vi "_PC_Pub_check_numstr.vi"(4 "ValueType":enum16{"Double", "Unsign Int32", "Sign Int32"}(ring), 7 "NumStringIn":string) -> (0 "DBL output":dbl, 1 "I64 output":i64, 2 "Error?":bool, 3 "NumStringOut":string)   [LabVIEW 2018]
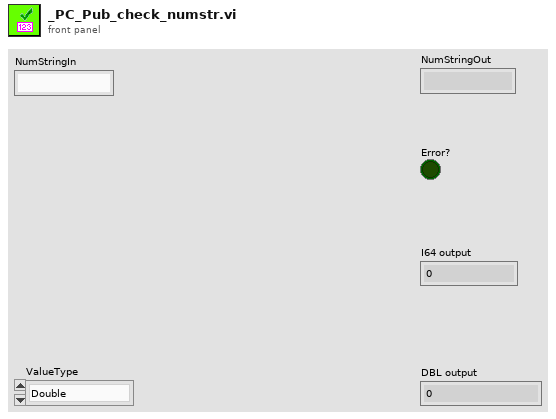
[diagram p1: front panel]
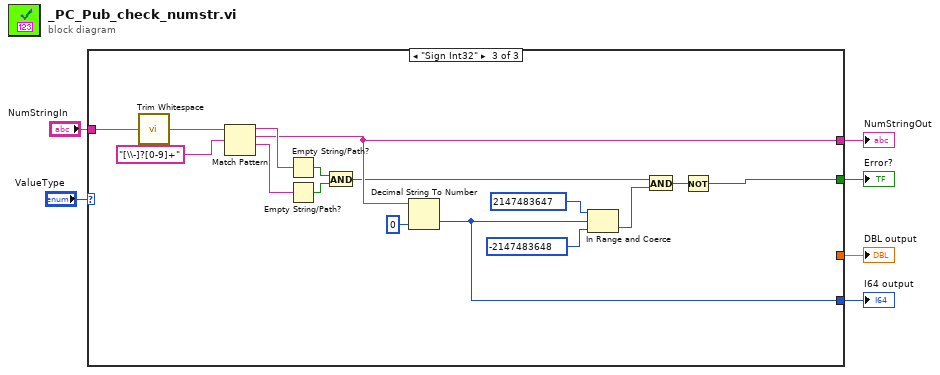
[diagram p0: block diagram]
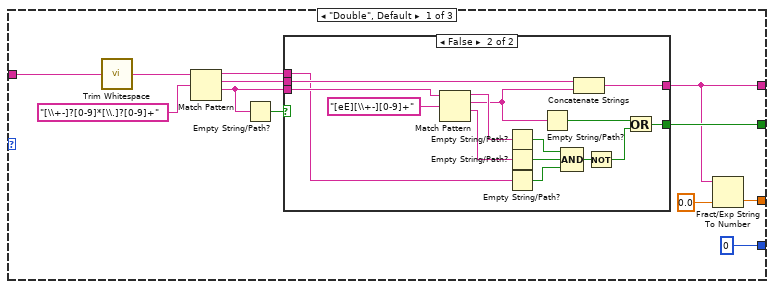
[diagram p2: hidden frame]
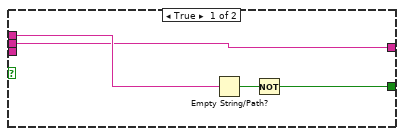
[diagram p3: hidden frame]
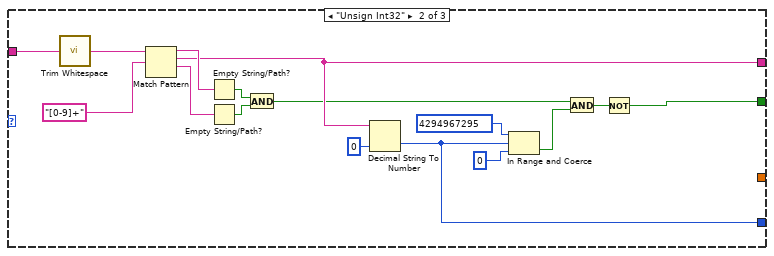
[diagram p4: hidden frame]
diagram:
  n1 = case shown="\"Sign Int32\"" "ValueType" {
    tunnel: "NumStringIn" -> [w12 w40 w56]
    tunnel: [w13 w41 w57] -> w5
    tunnel: [w10 w45 w61] -> w4
    tunnel: [i64 0 w38 w54] -> w2
    tunnel: [w8 _ _] -> w1
    frame "Double", Default {
      n2 = call <vilib>:"Trim Whitespace.vi"("string"=w12) -> ("trimmed string"=w11:string)  [unwired: 1 in]
      n3 = Match Pattern(string=w11, regular expression="[\\+-]?[0-9]*[\\.]?[0-9]+") -> (before substring=w14:string, match substring=w16:string, after substring=w15:string)  [unwired: 1 in, 1 out]
      n4 = Empty String/Path?(string/path=w15) -> (empty?=w17:bool)
      n5 = case shown="False" w17 {
        tunnel: w16 -> [w21 w27]
        tunnel: w15 -> [_ w36]
        tunnel: w14 -> [w22 w24]
        tunnel: [w19 w28] -> w13
        tunnel: [w21 w25] -> w10
        frame True {
          n6 = Empty String/Path?(string/path=w22) -> (empty?=w20:bool)
          n7 = Not(x=w20) -> (.not. x?=w19:bool)
        }
        frame False {
          n8 = Match Pattern(string=w36, regular expression="[eE][\\+-][0-9]+") -> (before substring=w34:string, match substring=w26:string, after substring=w35:string)  [unwired: 1 in, 1 out]
          n9 = Empty String/Path?(string/path=w34) -> (empty?=w33:bool)
          n10 = Empty String/Path?(string/path=w35) -> (empty?=w32:bool)
          n11 = Empty String/Path?(string/path=w24) -> (empty?=w23:bool)
          n12 = Empty String/Path?(string/path=w26) -> (empty?=w30:bool)
          n13 = Compound Arithmetic op=AND(w33, w32, w23) -> (w31:bool)
          n14 = Concatenate Strings(w27, w26) -> (w25:string)
          n15 = Not(x=w31) -> (.not. x?=w29:bool)
          n16 = Or(x=w30, y=w29) -> (x .or. y?=w28:bool)
        }
      }
      n17 = Fract/Exp String To Number(string=w10, default (0 dbl)=0.0) -> (number=w8:dbl)  [unwired: 2 in, 1 out]
    }
    frame "Unsign Int32" {
      n18 = call <vilib>:"Trim Whitespace.vi"("string"=w40) -> ("trimmed string"=w39:string)  [unwired: 1 in]
      n19 = Match Pattern(string=w39, regular expression="[0-9]+") -> (before substring=w51:string, match substring=w45:string, after substring=w52:string)  [unwired: 1 in, 1 out]
      n20 = Empty String/Path?(string/path=w51) -> (empty?=w49:bool)
      n21 = Empty String/Path?(string/path=w52) -> (empty?=w50:bool)
      n22 = And(x=w49, y=w50) -> (x .and. y?=w43:bool)
      n23 = Decimal String To Number(string=w45, default (0L)=u64 0 ("default (0 I32)")) -> (number=w38:u64)  [unwired: 1 in, 1 out]
      n24 = In Range and Coerce(upper limit=u32 4294967295, x=w38, lower limit=u32 0) -> (In Range?=w44:bool)  [unwired: 1 out]
      n25 = And(x=w43, y=w44) -> (x .and. y?=w42:bool)
      n26 = Not(x=w42) -> (.not. x?=w41:bool)
    }
    frame "Sign Int32" {
      n27 = call <vilib>:"Trim Whitespace.vi"("string"=w56) -> ("trimmed string"=w55:string)  [unwired: 1 in]
      n28 = Match Pattern(string=w55, regular expression="[\\-]?[0-9]+") -> (before substring=w67:string, match substring=w61:string, after substring=w68:string)  [unwired: 1 in, 1 out]
      n29 = Empty String/Path?(string/path=w67) -> (empty?=w65:bool)
      n30 = Empty String/Path?(string/path=w68) -> (empty?=w66:bool)
      n31 = And(x=w65, y=w66) -> (x .and. y?=w59:bool)
      n32 = Decimal String To Number(string=w61, default (0L)=i64 0 ("default (0 I32)")) -> (number=w54:i64)  [unwired: 1 in, 1 out]
      n33 = In Range and Coerce(upper limit=2147483647, x=w54, lower limit=-2147483648) -> (In Range?=w60:bool)  [unwired: 1 out]
      n34 = And(x=w59, y=w60) -> (x .and. y?=w58:bool)
      n35 = Not(x=w58) -> (.not. x?=w57:bool)
    }
  }
  "Error?" <- w5
  "NumStringOut" <- w4
  "I64 output" <- w2
  "DBL output" <- w1
